vi "fgv_pid_status.vi"(7 "cmd":T1, 8 "error in":errorcluster, 10 "pid dt":u32, 11 "pid output":dbl) -> (0 "error out":errorcluster, 2 "pid dt out":u32, 3 "pid output":dbl)   [LabVIEW 2019]
uses:
  Ctrl/pid-status.ctl
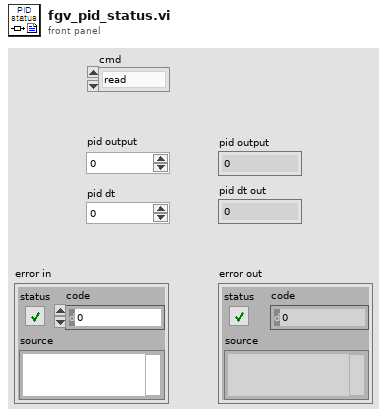
[diagram p1: front panel]
types:
  T1 = typedef "pid-status.ctl" = enum16{"read", "wirte pid dt", "wirte pid output"}
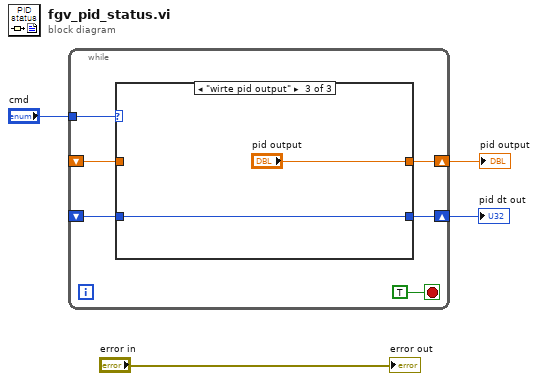
[diagram p0: block diagram]
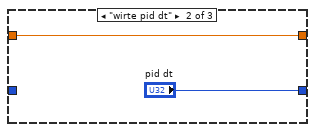
[diagram p3: hidden frame]
diagram:
  n1 = while {
    tunnel: "cmd" -> [w10]
    shift-right: [w8] -> w3
    shift-left: _ -> [w6]
    shift-right: [w7] -> w2
    shift-left: _ -> [w5]
    stop <- TRUE stop-if-true
    n2 = case shown="\"wirte pid output\"" w10 {
      tunnel: [w12 w13 "pid output"] -> w8
      tunnel: [w11 "pid dt" w15] -> w7
      tunnel: w6 -> [w12 w13 _]
      tunnel: w5 -> [w11 _ w15]
      frame "read", Default {
      }
      frame "wirte pid dt" {
      }
      frame "wirte pid output" {
      }
    }
  }
  "pid output" <- w3
  "pid dt out" <- w2
  "error out" <- "error in"
